vi "sphere tracking settings from scan settings.vi"(6 "gaussian":bool, 7 "sphere radius/sigma":u16, 8 "z-diff (um^2/ms)":dbl, 9 "Vdiff /(g^2*1ms)":dbl=0.01, 10 "lines per revolution":u16) -> (2 "tracking settings out":T1={"scan radius"=0, "2^16/lines per revolution"=1394, "gx"=0.0, "rtw"=0.0, "lines per revolution"=47, "vel diff"=0.0, "Dx - for pos only k-f"=0.0})   [LabVIEW 2010]
uses:
  FPGA tracking/polar tracking settings.ctl
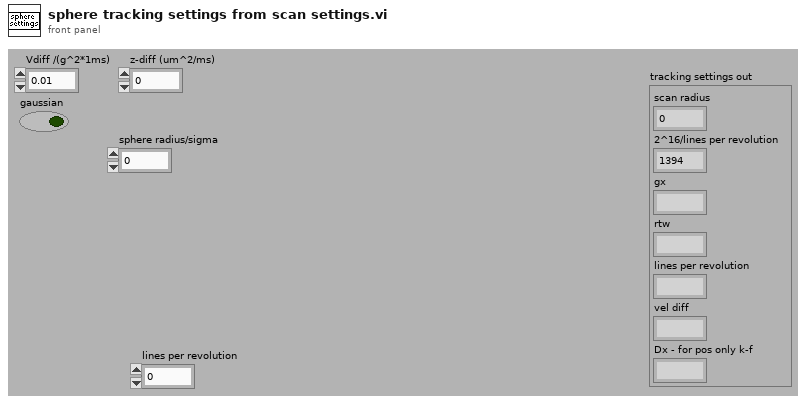
[diagram p1: front panel]
types:
  T1 = typedef "polar tracking settings.ctl" = cluster{"scan radius":u16, "2^16/lines per revolution":u16, "gx":fxp<+,16,8>, "rtw":fxp<+,16,26>, "lines per revolution":u8, "vel diff":fxp<+,24,-22>, "Dx - for pos only k-f":fxp<+,32,19>}
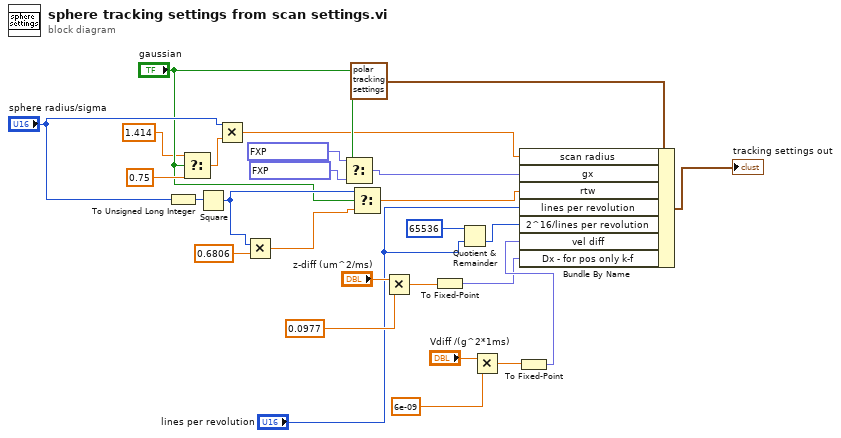
[diagram p0: block diagram]
diagram:
  n1 = To Unsigned Long Integer(number="sphere radius/sigma") -> (unsigned 32bit integer=w24:u32)
  n2 = Select(t=1.414, s="gaussian", f=0.75 ("y")) -> (s? t:f=w8:dbl)
  n3 = Square(x=w24) -> (x^2=w12:u32)
  n4 = Multiply(x="sphere radius/sigma", y=w8) -> (x*y=w6:dbl)
  n5 = Multiply(x=w12, y=0.6806) -> (x*y=w13:dbl)
  n6 = Select(t=fxp<+,16,8> 1.0, s="gaussian", f=fxp<+,16,8> 1.5546875 ("gx")) -> (s? t:f=w15:fxp<+,16,8>)
  n7 = Select(t=w12, s="gaussian", f=w13) -> (s? t:f=w11:dbl)
  n8 = Multiply(x="z-diff (um^2/ms)", y=0.0977) -> (x*y=w3:dbl)
  n9 = To Fixed-Point(number=w3) -> (fixed-point=w2:fxp<+,32,19>)  [unwired: 1 in]
  n10 = Quotient & Remainder(x=65536, y="lines per revolution") -> (floor(x/y)=w21:i32)  [unwired: 1 out]
  n11 = Multiply(x="Vdiff /(g^2*1ms)", y=6e-09) -> (x*y=w18:dbl)
  n12 = To Fixed-Point(number=w18) -> (fixed-point=w17:fxp<+,24,-22>)  [unwired: 1 in]
  n13 = Bundle By Name(cluster=T1 {"scan radius"=0, "2^16/lines per revolution"=1394, "gx"=0.0, "rtw"=0.0, "lines per revolution"=47, "vel diff"=0.0, "Dx - for pos only k-f"=0.0} ("tracking settings"), "scan radius"=w6, "gx"=w15, "rtw"=w11, "lines per revolution"="lines per revolution", "2^16/lines per revolution"=w21, "vel diff"=w17, "Dx - for pos only k-f"=w2) -> (→"tracking settings out":T1)
